vi "Read_From_NT_Into_Dashboard.vi"(1 "Values Array":string[](array[string]), 2 "Names Array":string[](array[string]), 3 "Pages":refnum<vi>[](array[refnum])) -> ()   [LabVIEW 2019]
doc: "This VI reads from NT tables that you input and writes it to the dash"
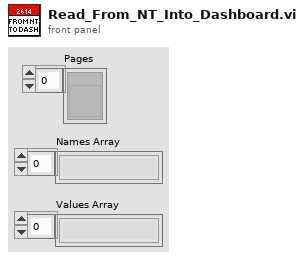
[diagram p1: front panel]
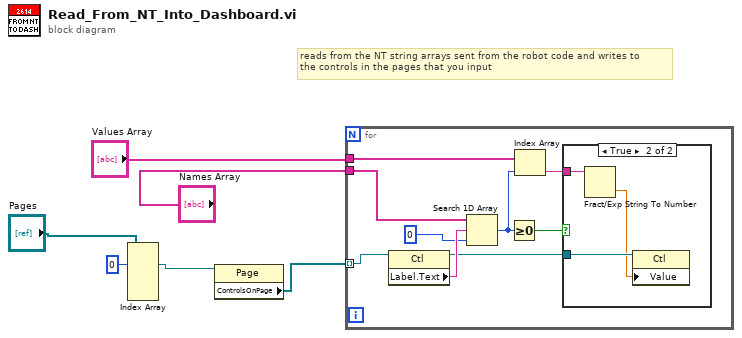
[diagram p0: block diagram]
diagram:
  # "reads from the NT string arrays sent from the robot code and writes to \nthe controls in the pages that you input"
  n1 = Index Array(array="Pages", index #1=0 ("index")) -> (element #1=w4:refnum<vi>)  [unwired: 4 in, 4 out]
  n2 = property class="Page"(reference=w4) -> ("ControlsOnPage"=w6:refnum<vi>[])  [unwired: 1 in, 2 out]
  n3 = for {
    tunnel: "Names Array" -> [w11]
    tunnel: "Values Array" -> [w8]
    tunnel: w6 -> [w7] mode=indexing
    n4 = property class="Ctl"(reference=w7) -> (reference out=w13:refnum<vi>, "Label.Text"=w15:string)  [unwired: 1 in, 1 out]
    n5 = Search 1D Array(1D array=w11, element=w15, start index (0)=0) -> (index of element=w10:i32)
    n6 = Greater Or Equal To 0?(x=w10) -> (x >= 0?=w12:bool)
    n7 = Index Array(array=w8, index=w10) -> (element=w9:string)
    n8 = case shown="True" w12 {
      tunnel: w13 -> [_ w18]
      tunnel: w9 -> [_ w16]
      frame False {
      }
      frame True {
        n9 = Fract/Exp String To Number(string=w16) -> (number=w17:dbl)  [unwired: 3 in, 1 out]
        n10 = property class="Ctl"(reference=w18, "Value"=w17) -> ()  [unwired: 1 in, 2 out]
      }
    }
  }
